vi "Requests.vi"(8 "error in (no error)":errorcluster, 9 "write enable":bool=TRUE, 11 "ICPCON PM-3112 in":refnum<class "ICPCON PM-3112-RTU.lvclass">) -> (0 "error out":errorcluster, 3 "ICPCON PM-3112 out":refnum<class "ICPCON PM-3112-RTU.lvclass">)   [LabVIEW 2021, in "ICPCON PM-3112-RTU.lvclass"]
uses:
  ICPCON PM-3112-RTU.lvclass
  D:/my_projects/projects/Algorithms/Labview/21/Master CR/Master CR.lvclass
  D:/my_projects/projects/Algorithms/Labview/21/Master CR/Devices/Serial/Serial.lvclass
  Master CR.lvclass/Master CR.ctl
  Modbus_v121c/Modbus Data Unit/Modbus Data Unit.lvclass/Modbus Data Unit.ctl
  Modbus_v121c/Network Protocol/Network Master/Network Master.lvclass/Network Master.ctl
  Network Protocol/Read Network Protocol.vi
  Modbus_v121c/Master Function Definition/Read Input Registers Request.vi
  Modbus_v121c/Master Function Definition/Read Input Registers Response.vi
  Modbus_v121c/Network Protocol/Network Master/Read write Master.vi
  Modbus_v121c/Modbus Data Unit/Construct PDU.vi
  Modbus_v121c/Utility/Bytes to U16s.vi
  Modbus_v121c/Master Function Definition/Function code mismatch error.vi
  Modbus_v121c/Data Model/Error Generator.vi
  Modbus_v121c/Modbus Data Unit/Deconstruct PDU.vi
  Serial/Serial.lvclass
  Modbus_v121c/Network Protocol/Network Master/Network Master.lvclass
  Modbus_v121c/Modbus Data Unit/Modbus Data Unit.lvclass
  Modbus_v121c/Data Model/Device Data Model.lvclass
  Modbus_v121c/Transmission Data Unit/Transmission Data Unit.lvclass
  Master CR.lvclass
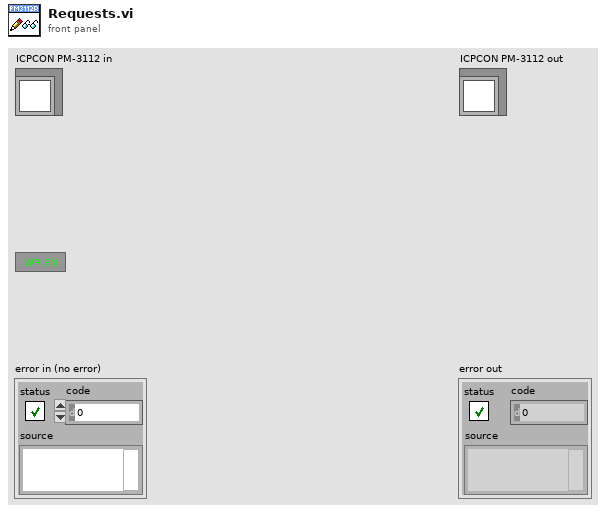
[diagram p1: front panel]
types:
  T1 = typedef "Device Data Model.lvclass/N channel.ctl" = cluster{"N DI channel":i32, "N DO channel":i32, "N AI channel":i32, "N AO channel":i32}
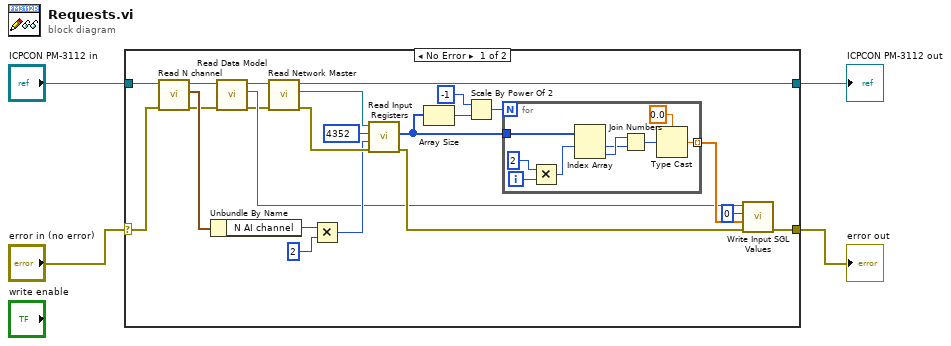
[diagram p0: block diagram]
diagram:
  n1 = case shown="No Error" "error in (no error)" {
    selector: "error in (no error)" -> [w22 w38]
    tunnel: [w19 w38] -> w1
    tunnel: [w15 w37] -> w2
    tunnel: "ICPCON PM-3112 in" -> [w24 w37]
    frame No Error {
      n2 = call "Read N channel.vi"("error in (no error)"=w22, "Master CR in"=w24) -> ("error out"=w21:errorcluster, "N channel"=w25:T1, "Master CR out"=w23:refnum<class "ICPCON PM-3112-RTU.lvclass">)  [unwired: 7 in]
      n3 = Unbundle By Name(w25) -> ("N AI channel"=w13:i32)
      n4 = call "Read Data Model.vi"("error in (no error)"=w21, "Master CR in"=w23) -> ("error out"=w5:errorcluster, "Data Model"=w6:refnum<class "Device Data Model.lvclass">, "Master CR out"=w18:refnum<class "ICPCON PM-3112-RTU.lvclass">)  [unwired: 7 in]
      n5 = call "Read Network Master.vi"("error in (no error)"=w5, "Serial in"=w18) -> ("error out"=w16:errorcluster, "Network Master"=w17:refnum<class "Network Master.lvclass">, "Serial out"=w15:refnum<class "ICPCON PM-3112-RTU.lvclass">)  [unwired: 7 in]
      n6 = Multiply(x=w13, y=2) -> (x*y=w14:i32)
      n7 = call "Read Input Registers.vi"("error in (no error)"=w16, "number of input registers"=w14, "starting address"=u16 4352, "Modbus master in"=w17) -> ("error out"=w20:errorcluster, "register values"=w8:u16[])  [unwired: 5 in, 1 out]
      n8 = Array Size(array=w8) -> (size(s)=w11:i32)
      n9 = Scale By Power Of 2(n=i16 -1, x=w11) -> (x*2^n=w9:i32)
      n10 = for {
        N: w9 -> [_]
        tunnel: w8 -> [w33]
        tunnel: [w31] -> w7 mode=indexing
        i -> [w36]
        n11 = Multiply(x=2 ("n"), y=w36) -> (x*y=w34:i32)
        n12 = Index Array(array=w33, index #1=w34) -> (element #1=w28:u16, element #2=w29:u16)  [unwired: 1 in]
        n13 = Join Numbers(hi=w29, lo=w28) -> ((hi.lo)=w30:u32)
        n14 = Type Cast(type=sgl 0.0 ("x"), x=w30) -> (*(type *) &x=w31:sgl)
      }
      n15 = call-dynamic "Write Input SGL Values.vi"("error in (no error)"=w20, "values"=w7, "starting address"=u16 0, "standard data model in"=w6) -> ("error out"=w19:errorcluster)  [unwired: 6 in, 1 out]
    }
    frame Error {
    }
  }
  "error out" <- w1
  "ICPCON PM-3112 out" <- w2
